vi "MAT read fixed test.vi"() -> ()   [LabVIEW 2020]
uses:
  MAT Type Representation.ctl
panel:
  out "error out":errorcluster
  out "cajk":bool
  in  "fmt list":T1
  out "Representation":T1
  in  "file path (use dialog)":path
  out "Matrix Name":string
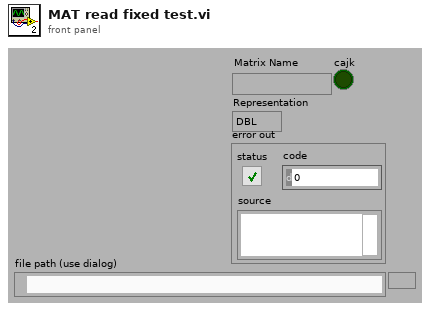
[diagram p1: front panel]
types:
  T1 = typedef "MAT Type Representation.ctl" = enum16{"DBL", "SGL", "I32", "I16", "U16", "U8", "CDB", "CSG", "STR"}
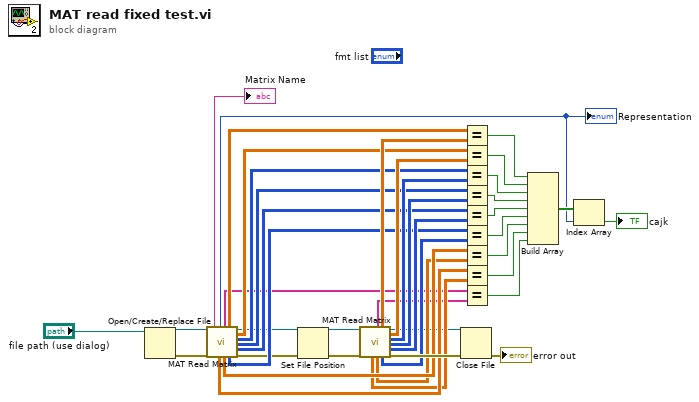
[diagram p0: block diagram]
diagram:
  n1 = Open/Create/Replace File(file path (use dialog)="file path (use dialog)") -> (refnum out=w40:refnum<file>, error out=w41:errorcluster)  [unwired: 5 in, 1 out]
  n2 = call "MAT Read Matrix.vi"("Ref Num"=w40, "Error In"=w41) -> ("Matrix Name"=→"Matrix Name":string, "Representation"=w8:T1, "CSG"=w22:csg[][], "STR"=w20:string[], "CDB"=w24:cdb[][], "DBL"=w36:dbl[][], "U8"=w26:u8[][], "Dup Ref Num"=w1:refnum<file>, "SGL"=w34:sgl[][], "I32"=w32:i32[][], "I16"=w30:i16[][], "U16"=w28:u16[][], "error out"=w4:errorcluster)  [unwired: 5 in]
  "Representation" <- w8
  n3 = Set File Position(refnum=w1, error in=w4) -> (refnum out=w2:refnum<file>, error out=w3:errorcluster)  [unwired: 2 in]
  n4 = call "MAT Read Matrix.vi"("Ref Num"=w2, "Error In"=w3) -> ("CSG"=w21:csg[][], "STR"=w19:string[], "CDB"=w23:cdb[][], "DBL"=w35:dbl[][], "U8"=w25:u8[][], "Dup Ref Num"=w6:refnum<file>, "SGL"=w33:sgl[][], "I32"=w31:i32[][], "I16"=w29:i16[][], "U16"=w27:u16[][], "error out"=w39:errorcluster)  [unwired: 5 in, 2 out]
  n5 = Close File(refnum=w6, error in=w39) -> (error out=→"error out":errorcluster)  [unwired: 1 out]
  n6 = Equal?(x=w36, y=w35) -> (x = y?=w18:bool)
  n7 = Equal?(x=w34, y=w33) -> (x = y?=w17:bool)
  n8 = Equal?(x=w32, y=w31) -> (x = y?=w16:bool)
  n9 = Equal?(x=w30, y=w29) -> (x = y?=w15:bool)
  n10 = Equal?(x=w28, y=w27) -> (x = y?=w14:bool)
  n11 = Equal?(x=w26, y=w25) -> (x = y?=w13:bool)
  n12 = Equal?(x=w24, y=w23) -> (x = y?=w12:bool)
  n13 = Equal?(x=w22, y=w21) -> (x = y?=w11:bool)
  n14 = Equal?(x=w20, y=w19) -> (x = y?=w10:bool)
  n15 = Build Array(w18, w17, w16, w15, w14, w13, w12, w11, w10) -> (w9:bool[])
  n16 = Index Array(array=w9, index=w8) -> (element=→"cajk":bool)
